vi "Update Controls.vi"(8 "error in (no error)":errorcluster, 11 "MHL References":T1) -> (0 "error out":errorcluster)   [LabVIEW 2015]
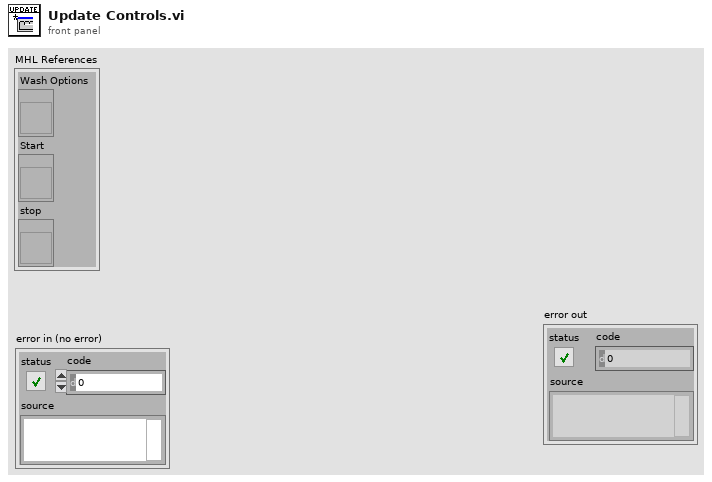
[diagram p1: front panel]
types:
  T1 = cluster{"Wash Options":refnum<vi>, "Start":refnum<vi>, "stop":refnum<vi>}
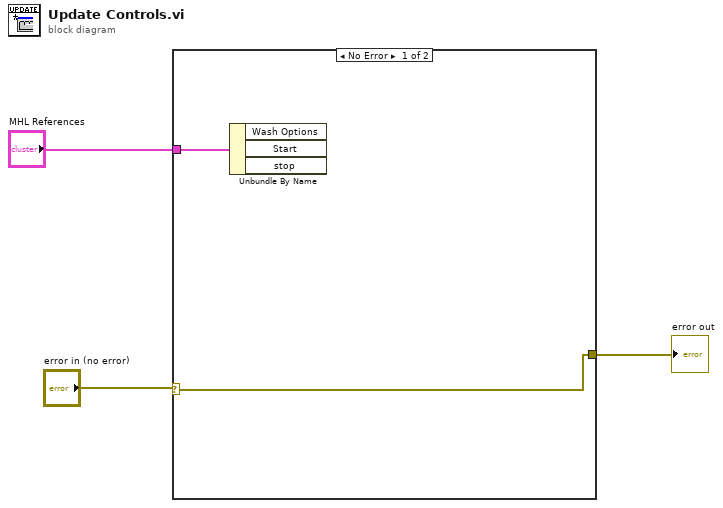
[diagram p0: block diagram]
diagram:
  n1 = case shown="No Error" "error in (no error)" {
    selector: "error in (no error)" -> [w5 w6]
    tunnel: [w5 w6] -> w2
    tunnel: "MHL References" -> [w4 _]
    frame No Error {
      n2 = Unbundle By Name(w4) -> ()  [unwired: 3 out]
    }
    frame Error {
    }
  }
  "error out" <- w2
